vi "3D Robot Frame.vi"(6 "wheel radius":dbl, 8 "error in (no error)":errorcluster, 10 "radius":dbl, 11 "name":string) -> (0 "error out":errorcluster, 3 "robot frame":refnum<vi>)   [LabVIEW 2015]
doc: "Creates the body object of the 3D mecanum robot."
uses:
  <vilib>/picture/3D Picture Control/Object/Create Object (name).vi
  <vilib>/picture/3D Picture Control/NI_3D Picture Control.lvlib
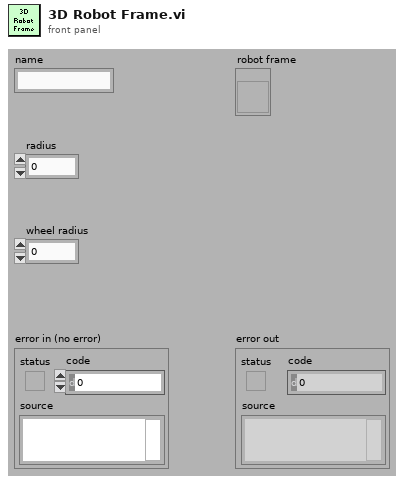
[diagram p1: front panel]
types:
  T1 = cluster{"Red":sgl, "Green":sgl, "Blue":sgl, "Alpha":sgl}
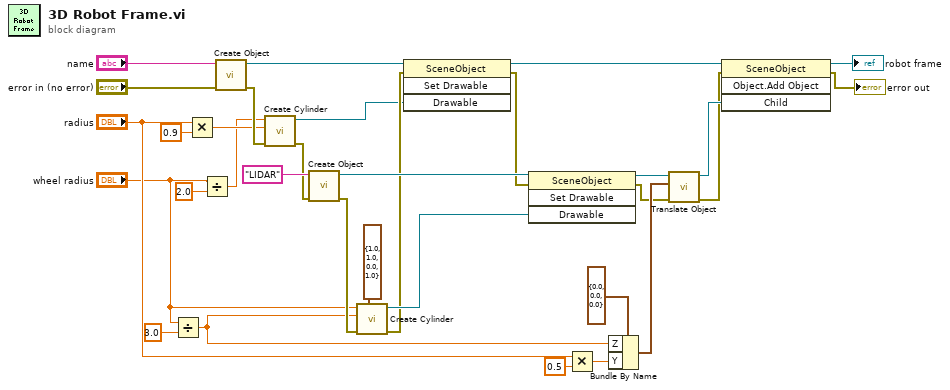
[diagram p0: block diagram]
diagram:
  n1 = Divide(x="wheel radius", y=3.0) -> (x/y=w4:dbl)
  n2 = Multiply(x="radius", y=0.9) -> (x*y=w6:dbl)
  n3 = Divide(x="wheel radius", y=2.0) -> (x/y=w1:dbl)
  n4 = call-poly <vilib>:"Create Object.vi"("error in (no error)"="error in (no error)", "Name"="name") -> ("error out"=w8:errorcluster, "Scene:New Object"=w30:refnum<vi>)  [unwired: 8 in]
  n5 = call <vilib>:"Create Cylinder.vi"("error in (no error)"=w8, "Radius"=w6, "Height"=w1) -> ("error out"=w9:errorcluster, "New Cylinder Refnum"=w10:refnum<vi>)  [unwired: 7 in]
  n6 = call-poly <vilib>:"Create Object.vi"("error in (no error)"=w9, "Name"="LIDAR") -> ("error out"=w14:errorcluster, "Scene:New Object"=w29:refnum<vi>)  [unwired: 8 in]
  n7 = call <vilib>:"Create Cylinder.vi"("Color"=T1 {"Red"=1.0, "Green"=1.0, "Blue"=0.0, "Alpha"=1.0}, "error in (no error)"=w14, "Radius"=w4, "Height"="wheel radius") -> ("error out"=w13:errorcluster, "New Cylinder Refnum"=w27:refnum<vi>)  [unwired: 6 out]
  n8 = invoke class="SceneObject" method="Set Drawable"(reference=w30, error in=w13, "Drawable"=w10) -> (reference out=w23:refnum<vi>, error out=w17:errorcluster)  [unwired: 1 in, 2 out]
  n9 = invoke class="SceneObject" method="Set Drawable"(reference=w29, error in=w17, "Drawable"=w27) -> (reference out=w26:refnum<vi>, error out=w11:errorcluster)  [unwired: 1 in, 2 out]
  n10 = Multiply(x="radius", y=0.5) -> (x*y=w19:dbl)
  n11 = Bundle By Name(cluster=cluster{"X":sgl, "Y":sgl, "Z":sgl} {"X"=0.0, "Y"=0.0, "Z"=0.0} ("Translation"), "Z"=w4, "Y"=w19) -> (w24:cluster{"X":sgl, "Y":sgl, "Z":sgl})
  n12 = call <vilib>:"Translate Object.vi"("error in (no error)"=w11, "Translation"=w24, "Scene.Object In"=w26) -> ("error out"=w16:errorcluster, "Scene.Object Out"=w22:refnum<vi>)  [unwired: 7 out]
  n13 = invoke class="SceneObject" method="Object.Add Object"(reference=w23, error in=w16, "Child"=w22) -> (reference out=→"robot frame":refnum<vi>, error out=→"error out":errorcluster)  [unwired: 1 in, 2 out]
